vi "SessionActive.vi"() -> (2 "Active":u8, 3 "Active":bool)   [LabVIEW 2015]
doc: "Configures device parameters for an NI 5170/5171"
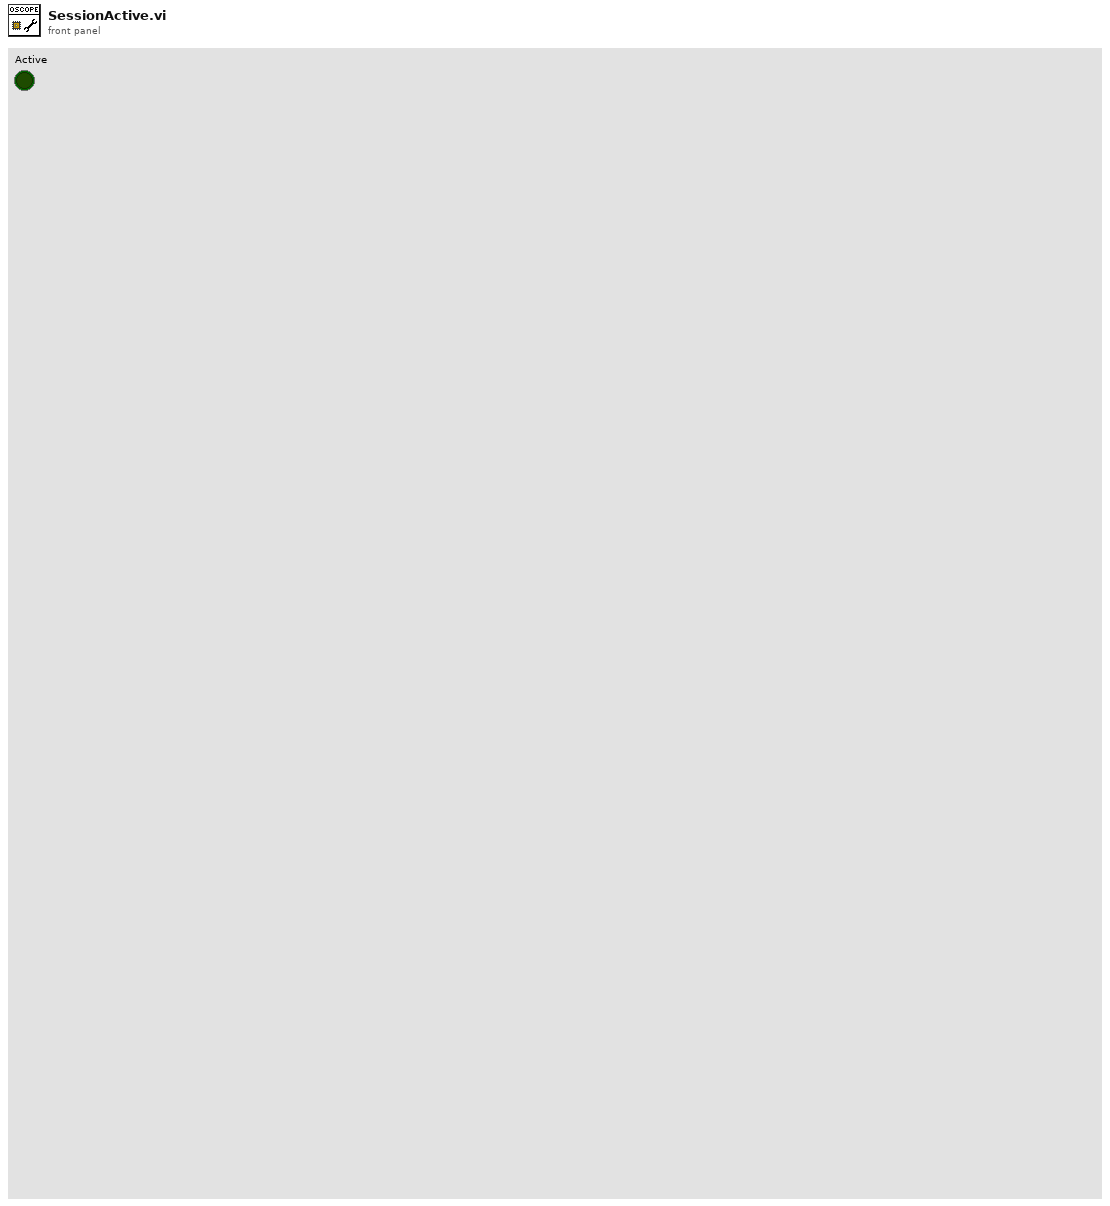
[diagram p1: front panel]
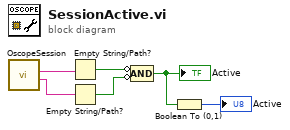
[diagram p0: block diagram]
diagram:
  n1 = call "OscopeSession.vi"() -> ("Bitfile Path Out"=w5:string, "Device Address Out"=w6:string)  [unwired: 9 in, 1 out]
  n2 = Empty String/Path?(string/path=w6) -> (empty?=w4:bool)
  n3 = Empty String/Path?(string/path=w5) -> (empty?=w3:bool)
  n4 = Compound Arithmetic op=AND(invert w4, invert w3) -> (w2:bool)
  "Active" <- w2
  n5 = Boolean To (0,1)(Boolean=w2) -> (0, 1=→"Active":i16)
